vi "activateDigitalFilter.vi"(6 "activate":bool=TRUE, 8 "error in (no error)":errorcluster, 9 "Med Filter type":T1, 10 "AVG Filter type":T2, 11 "State in":refnum<class "State.lvclass">) -> (0 "error out":errorcluster, 3 "State out":refnum<class "State.lvclass">)   [LabVIEW 2016, in "State.lvclass"]
uses:
  State.lvclass
  AVG Filter type.ctl
  MED Filter Type.ctl
  Electrometer.lvclass
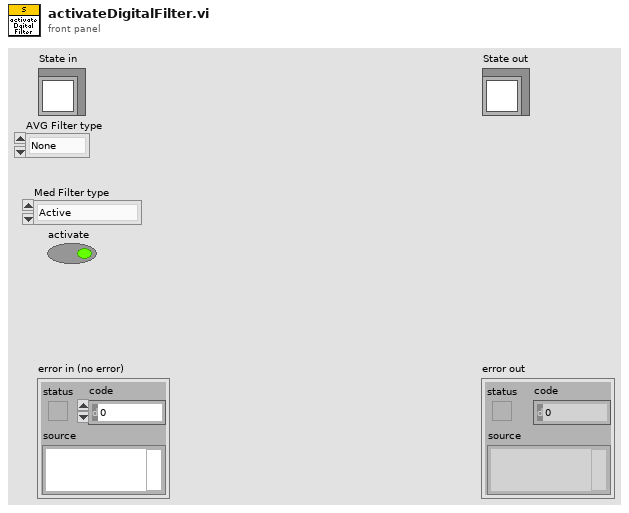
[diagram p1: front panel]
types:
  T1 = typedef "Electrometer.lvclass/MED Filter Type.ctl" = enum16{"Active", "None"}
  T2 = typedef "Electrometer.lvclass/AVG Filter type.ctl" = enum16{"None", "Scalar", "Advanced"}
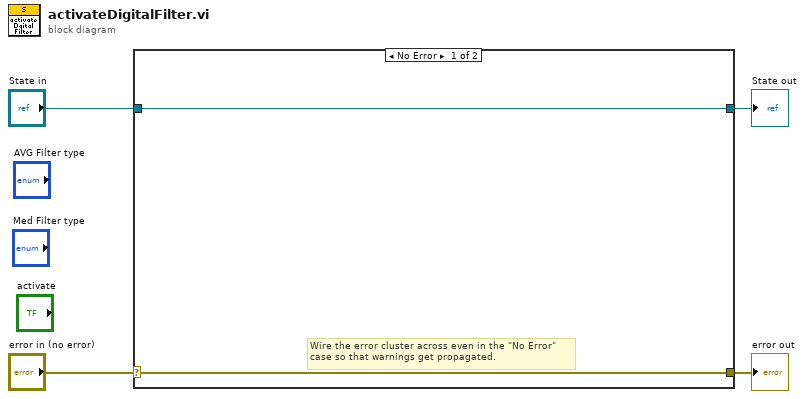
[diagram p0: block diagram]
diagram:
  n1 = case shown="No Error" "error in (no error)" {
    selector: "error in (no error)" -> [w5 w8]
    tunnel: [w5 w8] -> w3
    tunnel: [w6 w7] -> w1
    tunnel: "State in" -> [w6 w7]
    frame No Error {
      # "Wire the error cluster across even in the \"No Error\"\ncase so that warnings get propagated."
    }
    frame Error {
    }
  }
  "error out" <- w3
  "State out" <- w1
